vi "总磷氨氮插入数据.vi"(0 "table":string, 5 "data":T2={"时间标识"=timestamp(0 s since 1904-01-01), "测量模式"=enum."水样测试", "数据标记表"="N", "监测值"=0.0, "单位"=0, "数据标识"="", "因子编码"=0, "标样参考值"=0.0, "F0"=0.0, "F1"=0.0, "F2"=0.0, "F3"=0.0, "F4"=0.0, "F5"=0.0, "F6"=0.0, "F7"=0.0, "X"=0.0, "温度"=0.0, "湿度"=0.0, "量程标识"="", "SN"="", "跨度值"=0.0, "X1"=0.0} {"单位" items=["μg/L", "mg/L", "ppm", "mg/m3", "cm", "ppb", "μg/m3", "%", "nmol/mol", "μmol/mol", "MPN/L", "MPN/100ml", "ng/m3", "NTU", "无量纲", "ms/cm", "μs/cm"]}, 7 "关键参数":T1, 11 "error in (no error)":errorcluster) -> (15 "error out":errorcluster)   [LabVIEW 2016, in "斯坦道氨氮.lvlib"]
uses:
  <vilib>/Utility/error.llb/DialogType.ctl
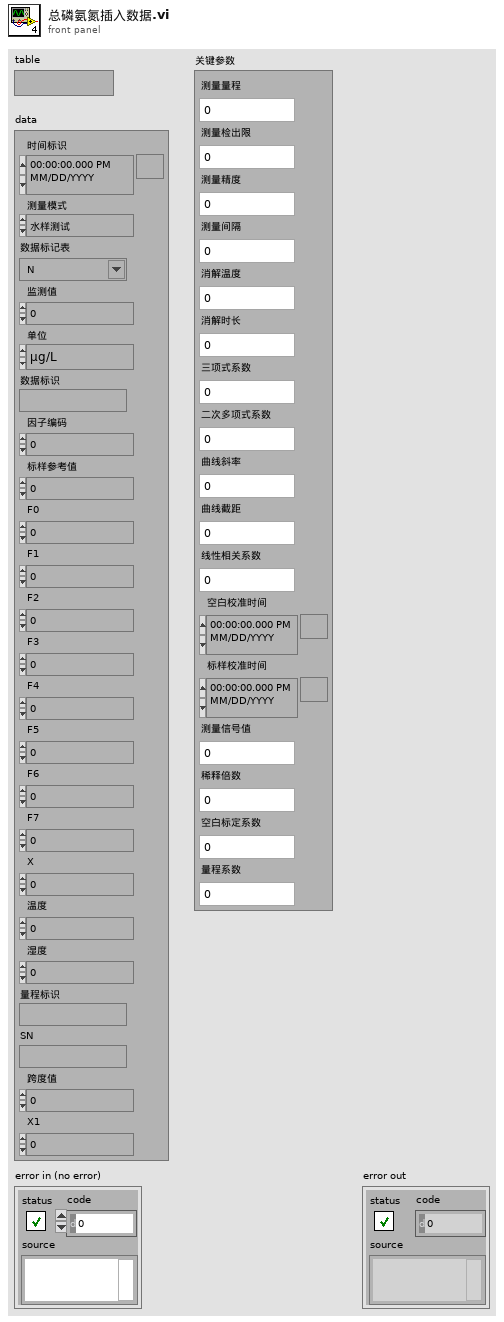
[diagram p1: front panel]
types:
  T1 = typedef "斯坦道氨氮.lvlib/关键参数.ctl" = cluster{"测量量程":sgl, "测量检出限":sgl, "测量精度":sgl, "测量间隔":sgl, "消解温度":sgl, "消解时长":sgl, "三项式系数":sgl, "二次多项式系数":sgl, "曲线斜率":sgl, "曲线截距":sgl, "线性相关系数":sgl, "空白校准时间":timestamp, "标样校准时间":timestamp, "测量信号值":sgl, "稀释倍数":sgl, "空白标定系数":sgl, "量程系数":sgl}
  T2 = cluster{"时间标识":timestamp, "测量模式":enum16{"维护数据", "水样测试", "标样核查", "零点核查", "跨度核查", "空白测试", "平行样测试", "加标回收", "空白校准", "标样校准", "初始化（清洗）", "快捷测试"}, "数据标记表":string, "监测值":sgl, "单位":u16, "数据标识":string, "因子编码":u32, "标样参考值":sgl, "F0":sgl, "F1":sgl, "F2":sgl, "F3":sgl, "F4":sgl, "F5":sgl, "F6":sgl, "F7":sgl, "X":sgl, "温度":sgl, "湿度":sgl, "量程标识":string, "SN":string, "跨度值":sgl, "X1":sgl}
  T3 = typedef "DialogType.ctl" = u16
  T4 = typedef "营养盐字段定义.ctl" = cluster{"时间":timestamp, "测量模式":string, "数据类型":string, "检测值":sgl, "单位":string, "数据标识":string, "X":sgl, "量程标识":string, "SN":string, "标样参考值":sgl, "跨度值":sgl, "F0":sgl, "F1":sgl, "F2":sgl, "F3":sgl, "F4":sgl, "F5":sgl, "F6":sgl, "F7":sgl, "X1":sgl, "因子编码":string, "温度":sgl, "湿度":sgl, "测量量程":sgl, "测量检出限":sgl, "测量精度":sgl, "测量间隔":sgl, "消解温度":sgl, "消解时长":sgl, "三项式系数":sgl, "二次多项式系数":sgl, "曲线斜率":sgl, "曲线截距":sgl, "线性相关系数":sgl, "空白校准时间":timestamp, "标样校准时间":timestamp, "测量信号值":sgl, "稀释倍数":sgl, "空白标定系数":sgl, "量程系数":sgl, "LastTime":timestamp}
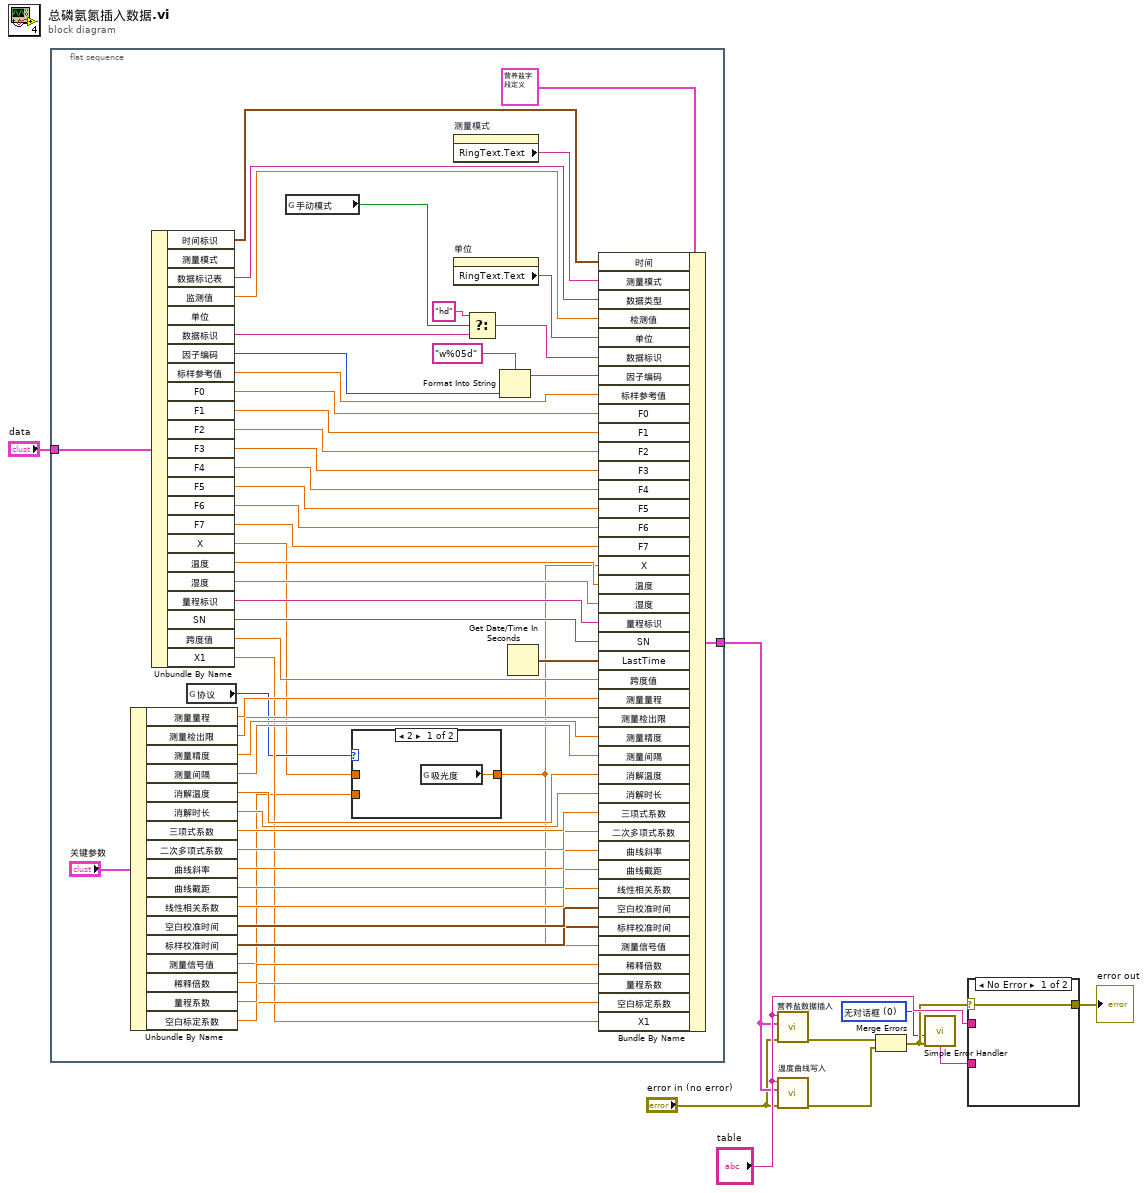
[diagram p0: block diagram]
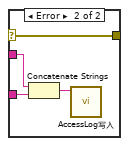
[diagram p3: hidden frame]
diagram:
  w2 = T3 0 items=["无对话框", "确定信息", "继续或停止信息", "确定信息＋警告", "继续/停止+警告"] ("type of dialog (OK msg:1)")
  n1 = flat-sequence {
    tunnel: "data" -> [w43]
    tunnel: [w19] -> w6
    frame #0 {
      n2 = Unbundle By Name("关键参数") -> ("测量量程"=w37:sgl, "测量检出限"=w36:sgl, "测量精度"=w35:sgl, "测量间隔"=w34:sgl, "消解温度"=w33:sgl, "消解时长"=w32:sgl, "三项式系数"=w31:sgl, "二次多项式系数"=w30:sgl, "曲线斜率"=w29:sgl, "曲线截距"=w28:sgl, "线性相关系数"=w27:sgl, "空白校准时间"=w26:timestamp, "标样校准时间"=w25:timestamp, "测量信号值"=w12:sgl, "稀释倍数"=w24:sgl, "量程系数"=w23:sgl, "空白标定系数"=w22:sgl)
      n3 = Unbundle By Name(w43) -> ("时间标识"=w62:timestamp, "数据标记表"=w60:string, "监测值"=w59:sgl, "数据标识"=w16:string, "因子编码"=w42:u32, "标样参考值"=w57:sgl, "F0"=w56:sgl, "F1"=w55:sgl, "F2"=w54:sgl, "F3"=w53:sgl, "F4"=w52:sgl, "F5"=w51:sgl, "F6"=w50:sgl, "F7"=w49:sgl, "X"=w13:sgl, "温度"=w48:sgl, "湿度"=w47:sgl, "量程标识"=w46:string, "SN"=w45:string, "跨度值"=w39:sgl, "X1"=w21:sgl)  [unwired: 2 out]
      n4 = global read "总磷总氮断电保存全局变量.vi" "协议"() -> (w14:u16)
      n5 = global read "VAR总磷总氮全局变量.vi" "手动模式"() -> (w18:bool)
      n6 = case shown="2" w14 {
        tunnel: w13 -> [_ w64]
        tunnel: [w63 w64] -> w11
        tunnel: w12 -> [_ _]
        frame 2 {
          n7 = global read "总磷总氮断电保存全局变量.vi" "吸光度"() -> (w63:sgl)
        }
        frame 1, Default {
        }
      }
      n8 = property on="测量模式" class="Enum (strict)"() -> ("RingText.Text"=w61:string)  [unwired: 2 in, 2 out]
      n9 = property on="单位" class="Ring (strict)"() -> ("RingText.Text"=w58:string)  [unwired: 2 in, 2 out]
      n10 = Select(t="hd", s=w18, f=w16) -> (s? t:f=w15:string)
      n11 = Format Into String(format string="w%05d" ("格式字符串"), w42) -> (resulting string=w40:string)  [unwired: 2 in, 1 out]
      n12 = Get Date/Time In Seconds() -> (seconds since 1Jan1904=w44:timestamp)
      n13 = Bundle By Name(cluster=T4 {"时间"=timestamp(0 s since 1904-01-01), "测量模式"="水样测试", "数据类型"="N", "检测值"=0.0, "单位"="mg/L", "数据标识"="N", "X"=0.0, "量程标识"="", "SN"="", "标样参考值"=0.0, "跨度值"=0.0, "F0"=0.0, "F1"=0.0, "F2"=0.0, "F3"=0.0, "F4"=0.0, "F5"=0.0, "F6"=0.0, "F7"=0.0, "X1"=0.0, "因子编码"="", "温度"=0.0, "湿度"=0.0, "测量量程"=0.0, "测量检出限"=0.0, "测量精度"=0.0, "测量间隔"=0.0, "消解温度"=0.0, "消解时长"=0.0, "三项式系数"=0.0, "二次多项式系数"=0.0, "曲线斜率"=0.0, "曲线截距"=0.0, "线性相关系数"=0.0, "空白校准时间"=timestamp(0 s since 1904-01-01), "标样校准时间"=timestamp(0 s since 1904-01-01), "测量信号值"=0.0, "稀释倍数"=0.0, "空白标定系数"=0.0, "量程系数"=0.0, "LastTime"=timestamp(0 s since 1904-01-01)} ("data"), "时间"=w62, "测量模式"=w61, "数据类型"=w60, "检测值"=w59, "单位"=w58, "数据标识"=w15, "因子编码"=w40, "标样参考值"=w57, "F0"=w56, "F1"=w55, "F2"=w54, "F3"=w53, "F4"=w52, "F5"=w51, "F6"=w50, "F7"=w49, "X"=w11, "温度"=w48, "湿度"=w47, "量程标识"=w46, "SN"=w45, "LastTime"=w44, "跨度值"=w39, "测量量程"=w37, "测量检出限"=w36, "测量精度"=w35, "测量间隔"=w34, "消解温度"=w33, "消解时长"=w32, "三项式系数"=w31, "二次多项式系数"=w30, "曲线斜率"=w29, "曲线截距"=w28, "线性相关系数"=w27, "空白校准时间"=w26, "标样校准时间"=w25, "测量信号值"=w11, "稀释倍数"=w24, "量程系数"=w23, "空白标定系数"=w22, "X1"=w21) -> (w19:T4)
    }
  }
  n14 = call "营养盐数据插入.vi"("Tabe Name"="table", "data"=w6, "错误输入（无错误）"="error in (no error)") -> ("错误输出"=w8:errorcluster)  [unwired: 7 in]
  n15 = call "温度曲线写入.vi"("error in (no error)"="error in (no error)", "columns"=w6, "table"="table") -> ("错误输出"=w4:errorcluster)  [unwired: 8 in]
  n16 = Merge Errors(w8, w4) -> (w3:errorcluster)
  n17 = call <vilib>:"Simple Error Handler.vi"("type of dialog (OK msg:1)"=w2, "error in (no error)"=w3) -> ("message"=w1:string)  [unwired: 3 in, 4 out]
  n18 = case shown="No Error" w3 {
    selector: w3 -> [w65 w69]
    tunnel: [w65 w69] -> w10
    tunnel: "table" -> [_ w68]
    tunnel: w1 -> [_ w67]
    frame No Error {
    }
    frame Error {
      n19 = Concatenate Strings(w68, w67) -> (w66:string)
      n20 = call "AccessLog写入.vi"("Log"=w66) -> ()  [unwired: 11 in]
    }
  }
  "error out" <- w10
